vi "YAFTAF_ClassCast.vi"(11 "LocalIn":refnum<class>) -> (3 "LocalOut":refnum<class "YAFTAF.lvclass">)   [LabVIEW 2021, in "YAFTAF.lvclass"]
uses:
  YAFTAF.lvclass
  YAFTAF.lvclass/YAFTAF.ctl
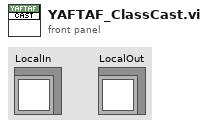
[diagram p1: front panel]
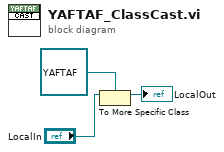
[diagram p0: block diagram]
diagram:
  n1 = To More Specific Class(target class=refnum<class "YAFTAF.lvclass"> refnum ("reference in"), reference="LocalIn") -> (specific class reference=→"LocalOut":refnum<class "YAFTAF.lvclass">)  [unwired: 1 in, 1 out]
